vi "Main On Compile VI_Get Decimation Ch Info.vi"(8 "error in (no error)":errorcluster, 10 "Section Reference":T1 format="%.0x", 11 "Device Reference":T1 format="%.0x") -> (0 "error out":errorcluster, 3 "Decimation FIFO Index":i32)   [LabVIEW 2019, in "RefMem DMA System Explorer.lvlib"]
uses:
  <vilib>/NI VeriStand/Custom Device API/Custom Device Item Ref.ctl
  RefMem DMA System Explorer.lvlib
  <vilib>/NI VeriStand/Custom Device Tools/Custom Device Utility Library/Custom Device Utility Library.lvlib
  Shared/Constants.vi
  Shared/RefMem DMA Shared.lvlib
  <vilib>/NI VeriStand/Custom Device API/Custom Device API.lvlib
  <vilib>/NI VeriStand/Custom Device Tools/Custom Device Utility Library/NI VeriStand - Search for All Items by GUID.vi
  <vilib>/NI VeriStand/Custom Device Tools/Custom Device Utility Library/NI VeriStand - Search for Item by GUID.vi
  <vilib>/NI VeriStand/Custom Device API/Get Item Property (U32).vi
  <vilib>/NI VeriStand/Custom Device API/Get Item Property (U16).vi
panel:
  out "FIFO Index Decimation Table":i32[](array[numeric])=[0, 2, 2, 0, 3]
  out "Block Address decimation table":u32[](array[numeric])=[0, 2, 2, 0, 3]
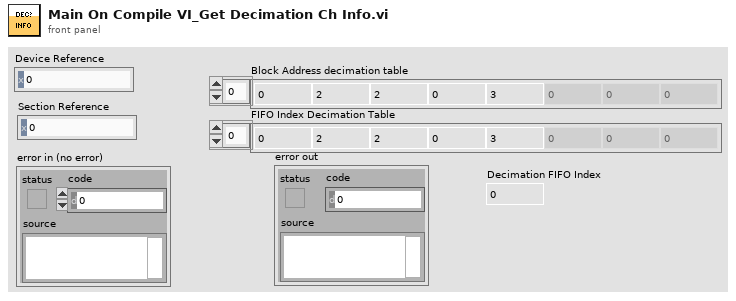
[diagram p1: front panel]
types:
  T1 = typedef "Custom Device API.lvlib/Custom Device Item Ref.ctl" = u64
  T2 = typedef "Custom Device API.lvlib/Custom Device Item Info.ctl" = cluster{"Name":string, "Is Channel":bool, "GUID":string, "Is Waveform":bool}
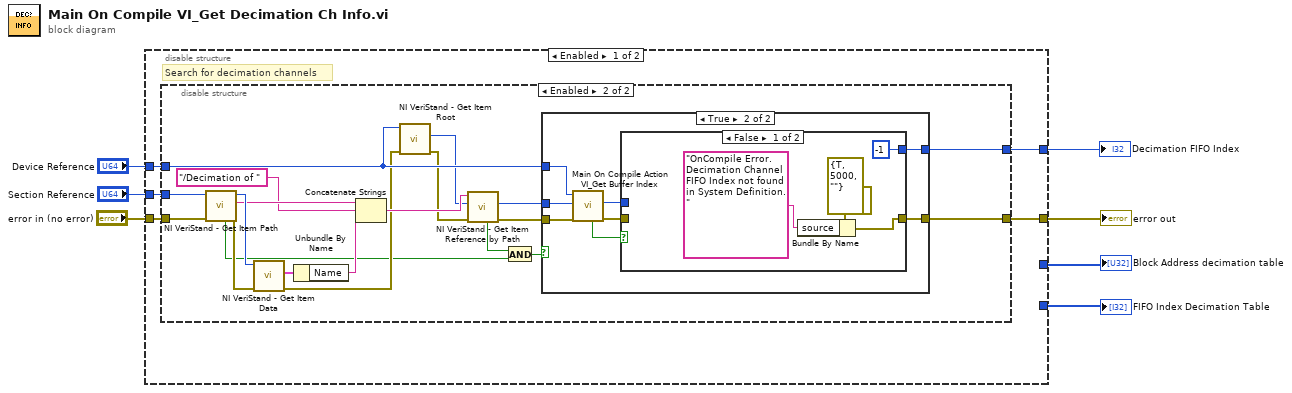
[diagram p0: block diagram]
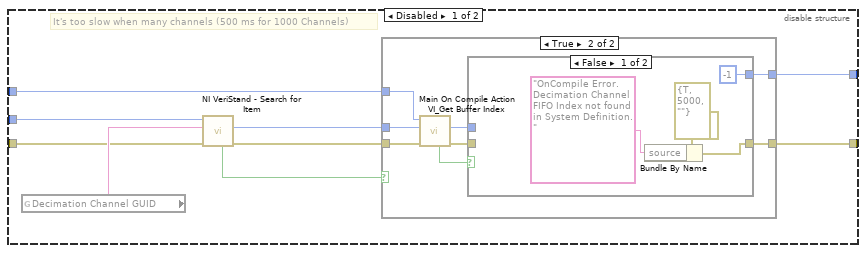
[diagram p2: hidden frame]
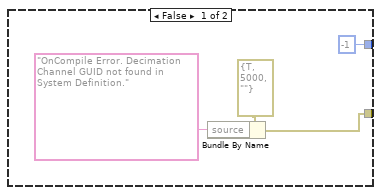
[diagram p3: hidden frame]
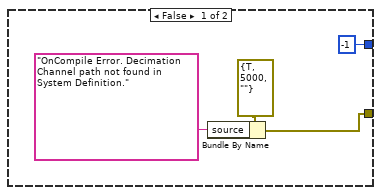
[diagram p5: hidden frame]
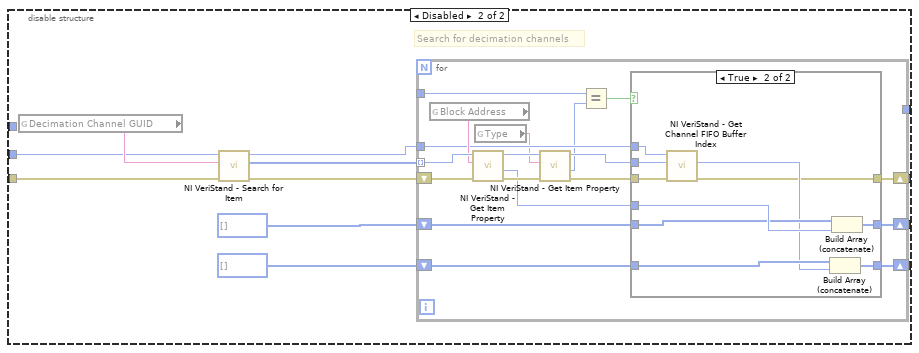
[diagram p7: hidden frame]
diagram:
  n1 = disable-structure shown="Enabled" {
    disable-tunnel: "error in (no error)" -> [w12 w83]
    disable-tunnel: "Section Reference" -> [w11 w82]
    disable-tunnel: [w8 w80] -> w5
    disable-tunnel: [_ w79] -> w4
    disable-tunnel: [_ w78] -> w3
    disable-tunnel: "Device Reference" -> [w10 _]
    disable-tunnel: [w9 _] -> w1
    frame Enabled {
      # "Search for decimation channels"
      n2 = disable-structure shown="Enabled" {
        disable-tunnel: w12 -> [w20 w56]
        disable-tunnel: w11 -> [w19 w57]
        disable-tunnel: w10 -> [w15 w47]
        disable-tunnel: [w14 w59] -> w9
        disable-tunnel: [w13 w58] -> w8
        frame Disabled {
          # "It's too slow when many channels (500 ms for 1000 Channels)"
          n3 = global read "Constants.vi" "Decimation Channel GUID"() -> (w21:string)
          n4 = call-poly <vilib>:"NI VeriStand - Search for Item.vi"("error in"=w20, "Item GUID"=w21, "Section Ref in"=w19) -> ("error out"=w17:errorcluster, "Item Ref"=w16:T1, "Found"=w18:bool)  [unwired: 5 in, 1 out]
          n5 = case shown="True" w18 {
            tunnel: w17 -> [_ w33]
            tunnel: w16 -> [_ w32]
            tunnel: w15 -> [_ w31]
            tunnel: [-1 ("Channel FIFO Buffer Index") w28] -> w14
            tunnel: [w24 w26] -> w13
            frame False {
              n6 = Bundle By Name(cluster=errorcluster {"status"=TRUE, "code"=5000, "source"=""} ("error out"), "source"="OnCompile Error. Decimation Channel GUID not found in System Definition." ("initial string")) -> (w24:errorcluster)
            }
            frame True {
              n7 = call "Main On Compile Action VI_Get Buffer Index.vi"("error in"=w33, "Channel Ref"=w32, "Device Ref in"=w31) -> ("error out"=w27:errorcluster, "Channel FIFO Buffer Index"=w29:i32, "Found"=w30:bool)  [unwired: 4 in, 2 out]
              n8 = case shown="False" w30 {
                tunnel: w29 -> [_ w39]
                tunnel: [-1 ("Channel FIFO Buffer Index") w39] -> w28
                tunnel: w27 -> [_ w38]
                tunnel: [w35 w38] -> w26
                frame False {
                  n9 = Bundle By Name(cluster=errorcluster {"status"=TRUE, "code"=5000, "source"=""} ("error out"), "source"="OnCompile Error. Decimation Channel FIFO Index not found in System Definition." ("initial string")) -> (w35:errorcluster)
                }
                frame True {
                }
              }
            }
          }
        }
        frame Enabled {
          n10 = call <vilib>:"NI VeriStand - Get Item Path.vi"("error in (no error)"=w56, "Item Ref in"=w57) -> ("error out"=w54:errorcluster, "Path"=w53:string, "Item Ref out"=w55:T1, "Found"=w40:bool)  [unwired: 6 in]
          n11 = call <vilib>:"NI VeriStand - Get Item Data.vi"("error in (no error)"=w54, "Item Ref in"=w55) -> ("error out"=w46:errorcluster, "Item Info"=w51:T2)  [unwired: 6 in, 2 out]
          n12 = Unbundle By Name(w51) -> ("Name"=w50:string)
          n13 = Concatenate Strings(w53, "/Decimation of " ("string"), w50) -> (w49:string)
          n14 = call <vilib>:"NI VeriStand - Get Item Root.vi"("error in (no error)"=w46, "Item Ref in"=w47) -> ("error out"=w45:errorcluster, "Root Ref out"=w44:T1)  [unwired: 6 in, 2 out]
          n15 = call <vilib>:"NI VeriStand - Get Item Reference by Path.vi"("error in (no error)"=w45, "Root Ref"=w44, "Item Path in"=w49) -> ("error out"=w48:errorcluster, "Item Ref"=w43:T1, "Found"=w41:bool)  [unwired: 5 in, 1 out]
          n16 = And(x=w41, y=w40) -> (x .and. y?=w42:bool)
          n17 = case shown="True" w42 {
            tunnel: w47 -> [_ w71]
            tunnel: [-1 ("Channel FIFO Buffer Index") w68] -> w59
            tunnel: [w62 w66] -> w58
            tunnel: w48 -> [_ w65]
            tunnel: w43 -> [_ w64]
            frame False {
              n18 = Bundle By Name(cluster=errorcluster {"status"=TRUE, "code"=5000, "source"=""} ("error out"), "source"="OnCompile Error. Decimation Channel path not found in System Definition." ("initial string")) -> (w62:errorcluster)
            }
            frame True {
              n19 = call "Main On Compile Action VI_Get Buffer Index.vi"("error in"=w65, "Channel Ref"=w64, "Device Ref in"=w71) -> ("error out"=w67:errorcluster, "Channel FIFO Buffer Index"=w69:i32, "Found"=w70:bool)  [unwired: 4 in, 2 out]
              n20 = case shown="False" w70 {
                tunnel: w69 -> [_ w77]
                tunnel: [-1 ("Channel FIFO Buffer Index") w77] -> w68
                tunnel: w67 -> [_ w76]
                tunnel: [w73 w76] -> w66
                frame False {
                  n21 = Bundle By Name(cluster=errorcluster {"status"=TRUE, "code"=5000, "source"=""} ("error out"), "source"="OnCompile Error. Decimation Channel FIFO Index not found in System Definition." ("initial string")) -> (w73:errorcluster)
                }
                frame True {
                }
              }
            }
          }
        }
      }
    }
    frame Disabled {
      # "Search for decimation channels"
      n22 = global read "Constants.vi" "Decimation Channel GUID"() -> (w84:string)
      n23 = call-poly <vilib>:"NI VeriStand - Search for Item.vi"("error in"=w83, "Item GUID"=w84, "Section Ref in"=w82) -> ("error out"=w88:errorcluster, "Item Refs"=w87:T1[], "Section Ref out"=w86:T1)  [unwired: 5 in, 1 out]
      n24 = for {
        tunnel: w86 -> [w104]
        tunnel: w87 -> [w107] mode=indexing
        shift-right: [w95] -> w78
        shift-left: i32[] [] ("Array") -> [w94]
        tunnel: [w97] -> w89
        shift-right: [w92] -> w79
        shift-left: u32[] [] ("Array") -> [w91]
        shift-right: [w90] -> w80
        shift-left: w88 -> [w106]
        n25 = global read "Constants.vi" "Block Address"() -> (w105:string)
        n26 = call-poly <vilib>:"NI VeriStand - Get Item Property.vi"("error in (no error)"=w106, "Property Name"=w105, "Item Ref in"=w107) -> ("error out"=w102:errorcluster, "Value"=w93:u32, "Item Ref out"=w103:T1)  [unwired: 5 in, 1 out]
        n27 = global read "Constants.vi" "Type"() -> (w99:string)
        n28 = call-poly <vilib>:"NI VeriStand - Get Item Property.vi"("error in (no error)"=w102, "Property Name"=w99, "Item Ref in"=w103) -> ("error out"=w101:errorcluster, "Value"=w98:u16, "Item Ref out"=w100:T1)  [unwired: 5 in, 1 out]
        n29 = Equal?(x=w97, y=w98) -> (x = y?=w96:bool)
        n30 = case shown="True" w96 {
          tunnel: w101 -> [w108 w120]
          tunnel: w104 -> [_ w119]
          tunnel: w100 -> [_ w118]
          tunnel: [w110 w113] -> w95
          tunnel: w94 -> [w110 w114]
          tunnel: w93 -> [_ w117]
          tunnel: [w109 w115] -> w92
          tunnel: w91 -> [w109 w116]
          tunnel: [w108 w111] -> w90
          frame False {
          }
          frame True {
            n31 = call <vilib>:"NI VeriStand - Get Channel FIFO Buffer Index.vi"("error in"=w120, "Channel Ref"=w118, "Device Ref in"=w119) -> ("error out"=w111:errorcluster, "Channel FIFO Buffer Index"=w112:i32)  [unwired: 4 in, 3 out]
            n32 = Build Array (concatenate)(w114, w112) -> (w113:i32[])
            n33 = Build Array (concatenate)(w116, w117) -> (w115:u32[])
          }
        }
      }
    }
  }
  "Block Address decimation table" <- w4
  "FIFO Index Decimation Table" <- w3
  "error out" <- w5
  "Decimation FIFO Index" <- w1
